vi "RGA_scan.vi"() -> ()   [LabVIEW 2017]
panel:
  in  "Number of Scans":string
  in  "Detector Index":string
  in  "E Gain Index":string
  in  "Source Index":string
  in  "Accuracy":string
  in  "Points per peak":string
  in  "End Mass":string
  in  "Measurement Name":string="test"
  in  "Start Mass":string
  out "standard error":string
  out "error out":errorcluster
  out "standard output":string
  out "return code":i32
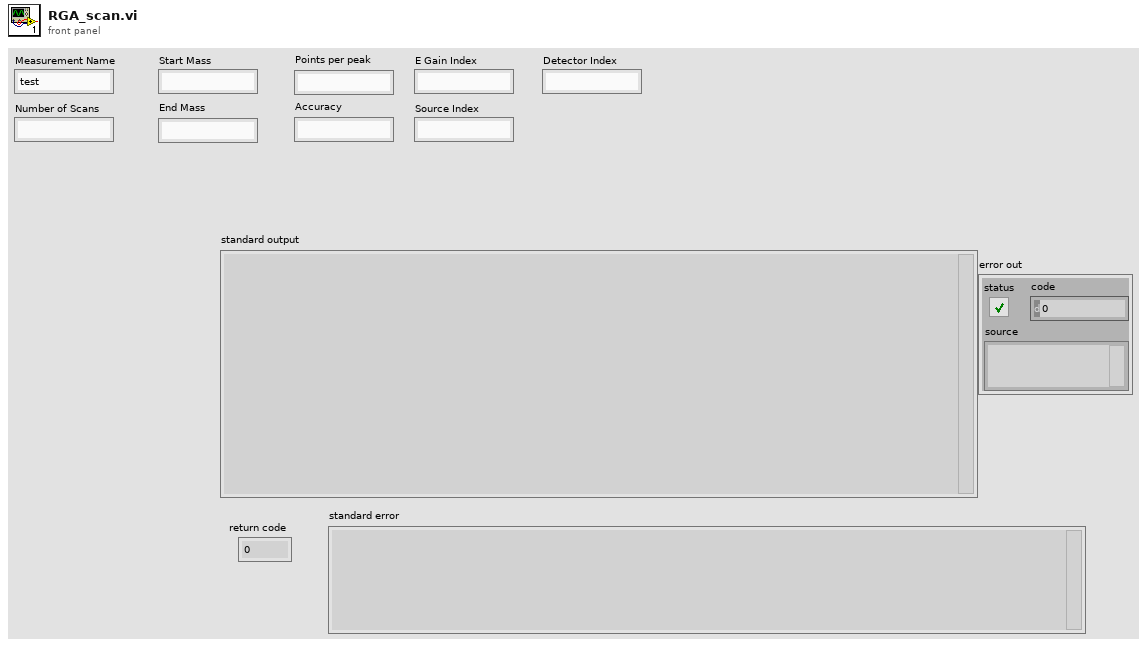
[diagram p1: front panel]
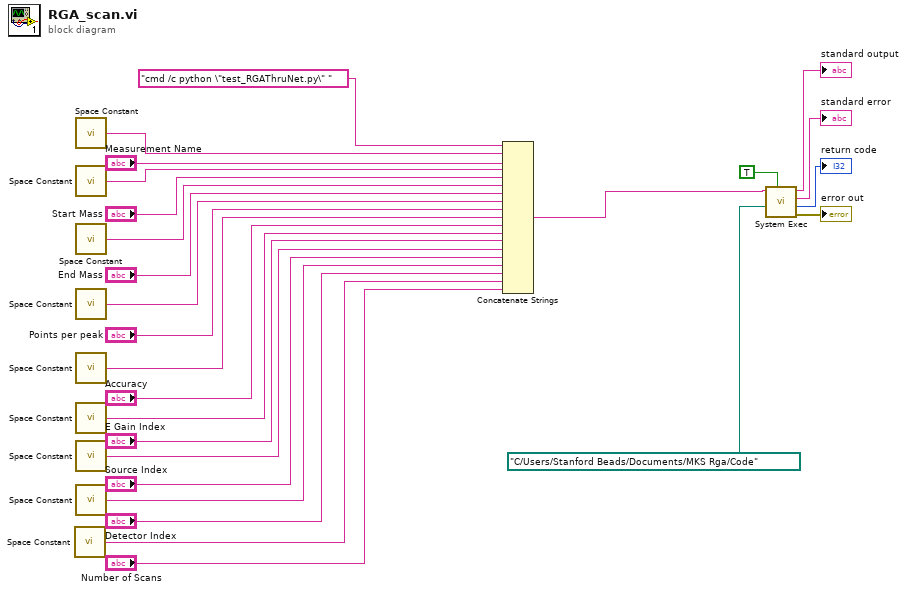
[diagram p0: block diagram]
diagram:
  n1 = call <vilib>:"Space Constant.vi"() -> ("String"=w2:string)
  n2 = call <vilib>:"Space Constant.vi"() -> ("String"=w19:string)
  n3 = call <vilib>:"Space Constant.vi"() -> ("String"=w17:string)
  n4 = call <vilib>:"Space Constant.vi"() -> ("String"=w15:string)
  n5 = call <vilib>:"Space Constant.vi"() -> ("String"=w7:string)
  n6 = call <vilib>:"Space Constant.vi"() -> ("String"=w8:string)
  n7 = call <vilib>:"Space Constant.vi"() -> ("String"=w6:string)
  n8 = call <vilib>:"Space Constant.vi"() -> ("String"=w5:string)
  n9 = call <vilib>:"Space Constant.vi"() -> ("String"=w4:string)
  n10 = Concatenate Strings("cmd /c python \"test_RGAThruNet.py\" " ("command line"), w19, "Measurement Name", w17, "Start Mass", w15, "End Mass", w7, "Points per peak", w8, "Accuracy", w6, "E Gain Index", w5, "Source Index", w4, "Detector Index", w2, "Number of Scans") -> (w3:string)
  n11 = call <vilib>:"System Exec.vi"("wait until completion? (T)"=TRUE, "working directory"=path "C:/Users/Stanford Beads/Documents/MKS Rga/Code", "command line"=w3) -> ("error out"=→"error out":errorcluster, "return code"=→"return code":i32, "standard error"=→"standard error":string, "standard output"=→"standard output":string)  [unwired: 5 in]
